vi "CellVolt181.vi"() -> ()   [LabVIEW 2018]
panel:
  in  "Boolean 15":bool
  in  "Boolean 14":bool
  in  "Boolean 13":bool
  in  "Boolean 12":bool
  in  "Table Control 15":string[][](table)=[["", "", "", "111"], ["", "", "", "112"], ["", "", "", "113"], ["", "", "", "114"], ["", "", "", "115"], ["", "", "", "116"], ["", "", "", "117"], ["", "", "", "118"], ["", "", "", "119"], ["", "", "", "120"], ["", "", "", "11"], ["", "", "", "12"], ["", "", "", "13"], ["", "", "", "14"], ["", "", "", "15"], ["", "", "", "16"], ["", "", "", "17"], ["", "", "", "18"], ["", "", "", "19"], ["", "", "", "20"], ["", "", "", "21"], ["", "", "", "22"], ["", "", "", "23"], ["", "", "", "24"]]
  in  "Table Control 14":string[][](table)=[["", "", "", "101"], ["", "", "", "102"], ["", "", "", "103"], ["", "", "", "104"], ["", "", "", "105"], ["", "", "", "106"], ["", "", "", "107"], ["", "", "", "108"], ["", "", "", "109"], ["", "", "", "110"], ["", "", "", "11"], ["", "", "", "12"], ["", "", "", "13"], ["", "", "", "14"], ["", "", "", "15"], ["", "", "", "16"], ["", "", "", "17"], ["", "", "", "18"], ["", "", "", "19"], ["", "", "", "20"], ["", "", "", "21"], ["", "", "", "22"], ["", "", "", "23"], ["", "", "", "24"]]
  in  "Table Control 13":string[][](table)=[["", "", "", "91"], ["", "", "", "92"], ["", "", "", "93"], ["", "", "", "94"], ["", "", "", "95"], ["", "", "", "96"], ["", "", "", "97"], ["", "", "", "98"], ["", "", "", "99"], ["", "", "", "100"], ["", "", "", "11"], ["", "", "", "12"], ["", "", "", "13"], ["", "", "", "14"], ["", "", "", "15"], ["", "", "", "16"], ["", "", "", "17"], ["", "", "", "18"], ["", "", "", "19"], ["", "", "", "20"], ["", "", "", "21"], ["", "", "", "22"], ["", "", "", "23"], ["", "", "", "24"]]
  in  "Table Control 12":string[][](table)=[["", "", "", "81"], ["", "", "", "82"], ["", "", "", "83"], ["", "", "", "84"], ["", "", "", "85"], ["", "", "", "86"], ["", "", "", "87"], ["", "", "", "88"], ["", "", "", "89"], ["", "", "", "90"], ["", "", "", "11"], ["", "", "", "12"], ["", "", "", "13"], ["", "", "", "14"], ["", "", "", "15"], ["", "", "", "16"], ["", "", "", "17"], ["", "", "", "18"], ["", "", "", "19"], ["", "", "", "20"], ["", "", "", "21"], ["", "", "", "22"], ["", "", "", "23"], ["", "", "", "24"]]
  in  "Table Control 11":string[][](table)=[["", "", "", "71"], ["", "", "", "72"], ["", "", "", "73"], ["", "", "", "74"], ["", "", "", "75"], ["", "", "", "76"], ["", "", "", "77"], ["", "", "", "78"], ["", "", "", "79"], ["", "", "", "80"], ["", "", "", "11"], ["", "", "", "12"], ["", "", "", "13"], ["", "", "", "14"], ["", "", "", "15"], ["", "", "", "16"], ["", "", "", "17"], ["", "", "", "18"], ["", "", "", "19"], ["", "", "", "20"], ["", "", "", "21"], ["", "", "", "22"], ["", "", "", "23"], ["", "", "", "24"]]
  in  "Boolean 10":bool
  in  "Boolean 9":bool
  in  "Boolean 8":bool
  in  "Boolean 7":bool
  in  "Boolean 6":bool
  in  "Boolean 5":bool
  in  "Table Control 10":string[][](table)=[["217"], ["218"], ["219"], ["220"], ["221"], ["222"], ["223"], ["224"], ["225"], ["226"], ["227"], ["228"], ["229"], ["230"], ["231"], ["232"], ["233"], ["234"], ["235"], ["236"], ["237"], ["238"], ["239"], ["240"]]
  in  "Table Control 9":string[][](table)=[["", "", "", "193", "", "", "", "", "", "", "193"], ["", "", "", "194", "", "", "", "", "", "", "194"], ["", "", "", "195", "", "", "", "", "", "", "195"], ["", "", "", "196", "", "", "", "", "", "", "196"], ["", "", "", "197", "", "", "", "", "", "", "197"], ["", "", "", "198", "", "", "", "", "", "", "198"], ["", "", "", "199", "", "", "", "", "", "", "199"], ["", "", "", "", "", "", "", "", "", "", "200"], ["", "", "", "", "", "", "", "", "", "", "201"], ["", "", "", "", "", "", "", "", "", "", "202"], ["", "", "", "", "", "", "", "", "", "", "203"], ["", "", "", "", "", "", "", "", "", "", "204"], ["", "", "", "", "", "", "", "", "", "", "205"], ["", "", "", "", "", "", "", "", "", "", "206"], ["", "", "", "", "", "", "", "", "", "", "207"], ["", "", "", "", "", "", "", "", "", "", "208"], ["", "", "", "", "", "", "", "", "", "", "209"], ["", "", "", "", "", "", "", "", "", "", "210"], ["", "", "", "", "", "", "", "", "", "", "211"], ["", "", "", "", "", "", "", "", "", "", "212"], ["", "", "", "", "", "", "", "", "", "", "213"], ["", "", "", "", "", "", "", "", "", "", "214"], ["", "", "", "", "", "", "", "", "", "", "215"], ["", "", "", "", "", "", "", "", "", "", "216"]]
  in  "Table Control 8":string[][](table)=[["", "", "", "169"], ["", "", "", "170"], ["", "", "", "171"], ["", "", "", "172"], ["", "", "", "173"], ["", "", "", "174"], ["", "", "", "175"], ["", "", "", "176"], ["", "", "", "177"], ["", "", "", "175"], ["", "", "", "179"], ["", "", "", "180"], ["", "", "", "181"], ["", "", "", "182"], ["", "", "", "183"], ["", "", "", "184"], ["", "", "", "185"], ["", "", "", "186"], ["", "", "", "187"], ["", "", "", "188"], ["", "", "", "189"], ["", "", "", "190"], ["", "", "", "191"], ["", "", "", "192"]]
  in  "Table Control 7":string[][](table)=[["", "", "", "145"], ["", "", "", "146"], ["", "", "", "147"], ["", "", "", "148"], ["", "", "", "149"], ["", "", "", "150"], ["", "", "", "151"], ["", "", "", "152"], ["", "", "", "153"], ["", "", "", "154"], ["", "", "", "155"], ["", "", "", "156"], ["", "", "", "157"], ["", "", "", "158"], ["", "", "", "159"], ["", "", "", "160"], ["", "", "", "161"], ["", "", "", "162"], ["", "", "", "163"], ["", "", "", "164"], ["", "", "", "165"], ["", "", "", "166"], ["", "", "", "167"], ["", "", "", "168"]]
  in  "Table Control 6":string[][](table)=[["", "", "", "121"], ["", "", "", "122"], ["", "", "", "123"], ["", "", "", "124"], ["", "", "", "125"], ["", "", "", "126"], ["", "", "", "127"], ["", "", "", "128"], ["", "", "", "129"], ["", "", "", "130"], ["", "", "", "131"], ["", "", "", "132"], ["", "", "", "133"], ["", "", "", "134"], ["", "", "", "135"], ["", "", "", "136"], ["", "", "", "137"], ["", "", "", "138"], ["", "", "", "139"], ["", "", "", "140"], ["", "", "", "141"], ["", "", "", "142"], ["", "", "", "143"], ["", "", "", "144"], ["", "", "", "145"]]
  in  "Table Control 5":string[][](table)=[["", "", "", "97"], ["", "", "", "98"], ["", "", "", "99"], ["", "", "", "100"], ["", "", "", "101"], ["", "", "", "102"], ["", "", "", "103"], ["", "", "", "104"], ["", "", "", "105"], ["", "", "", "106"], ["", "", "", "107"], ["", "", "", "108"], ["", "", "", "109"], ["", "", "", "110"], ["", "", "", "111"], ["", "", "", "112"], ["", "", "", "113"], ["", "", "", "114"], ["", "", "", "115"], ["", "", "", "116"], ["", "", "", "117"], ["", "", "", "118"], ["", "", "", "119"], ["", "", "", "120"]]
  in  "Table Control 4":string[][](table)=[["", "", "", "73"], ["", "", "", "74"], ["", "", "", "75"], ["", "", "", "76"], ["", "", "", "77"], ["", "", "", "78"], ["", "", "", "79"], ["", "", "", "80"], ["", "", "", "81"], ["", "", "", "82"], ["", "", "", "83"], ["", "", "", "84"], ["", "", "", "85"], ["", "", "", "86"], ["", "", "", "87"], ["", "", "", "88"], ["", "", "", "89"], ["", "", "", "90"], ["", "", "", "91"], ["", "", "", "92"], ["", "", "", "93"], ["", "", "", "94"], ["", "", "", "95"], ["", "", "", "96"], ["", "", "", "97"]]
  in  "Table Control 3":string[][](table)=[["", "", "", "49"], ["", "", "", "50"], ["", "", "", "51"], ["", "", "", "52"], ["", "", "", "53"], ["", "", "", "54"], ["", "", "", "55"], ["", "", "", "56"], ["", "", "", "57"], ["", "", "", "58"], ["", "", "", "59"], ["", "", "", "60"], ["", "", "", "61"], ["", "", "", "62"], ["", "", "", "63"], ["", "", "", "64"], ["", "", "", "65"], ["", "", "", "66"], ["", "", "", "67"], ["", "", "", "68"], ["", "", "", "69"], ["", "", "", "70"], ["", "", "", "71"], ["", "", "", "72"], ["", "", "", "73"]]
  in  "Table Control 2":string[][](table)=[["", "", "", "25"], ["", "", "", "26"], ["", "", "", "27"], ["", "", "", "28"], ["", "", "", "29"], ["", "", "", "30"], ["", "", "", "31"], ["", "", "", "32"], ["", "", "", "33"], ["", "", "", "34"], ["", "", "", "35"], ["", "", "", "36"], ["", "", "", "37"], ["", "", "", "38"], ["", "", "", "39"], ["", "", "", "40"], ["", "", "", "41"], ["", "", "", "42"], ["", "", "", "43"], ["", "", "", "44"], ["", "", "", "45"], ["", "", "", "46"], ["", "", "", "47"], ["", "", "", "48"]]
  in  "Table Control":string[][](table)=[["", "", "", "61"], ["", "", "", "62"], ["", "", "", "63"], ["", "", "", "64"], ["", "", "", "65"], ["", "", "", "66"], ["", "", "", "67"], ["", "", "", "68"], ["", "", "", "69"], ["", "", "", "70"], ["", "", "", "11"], ["", "", "", "12"], ["", "", "", "13"], ["", "", "", "14"], ["", "", "", "15"], ["", "", "", "16"], ["", "", "", "17"], ["", "", "", "18"], ["", "", "", "19"], ["", "", "", "20"], ["", "", "", "21"], ["", "", "", "22"], ["", "", "", "23"], ["", "", "", "24"]]
  in  "Boolean 4":bool
  in  "Boolean 3":bool
  in  "Boolean 2":bool
  in  "Boolean":bool
  # "BMS Monitor"
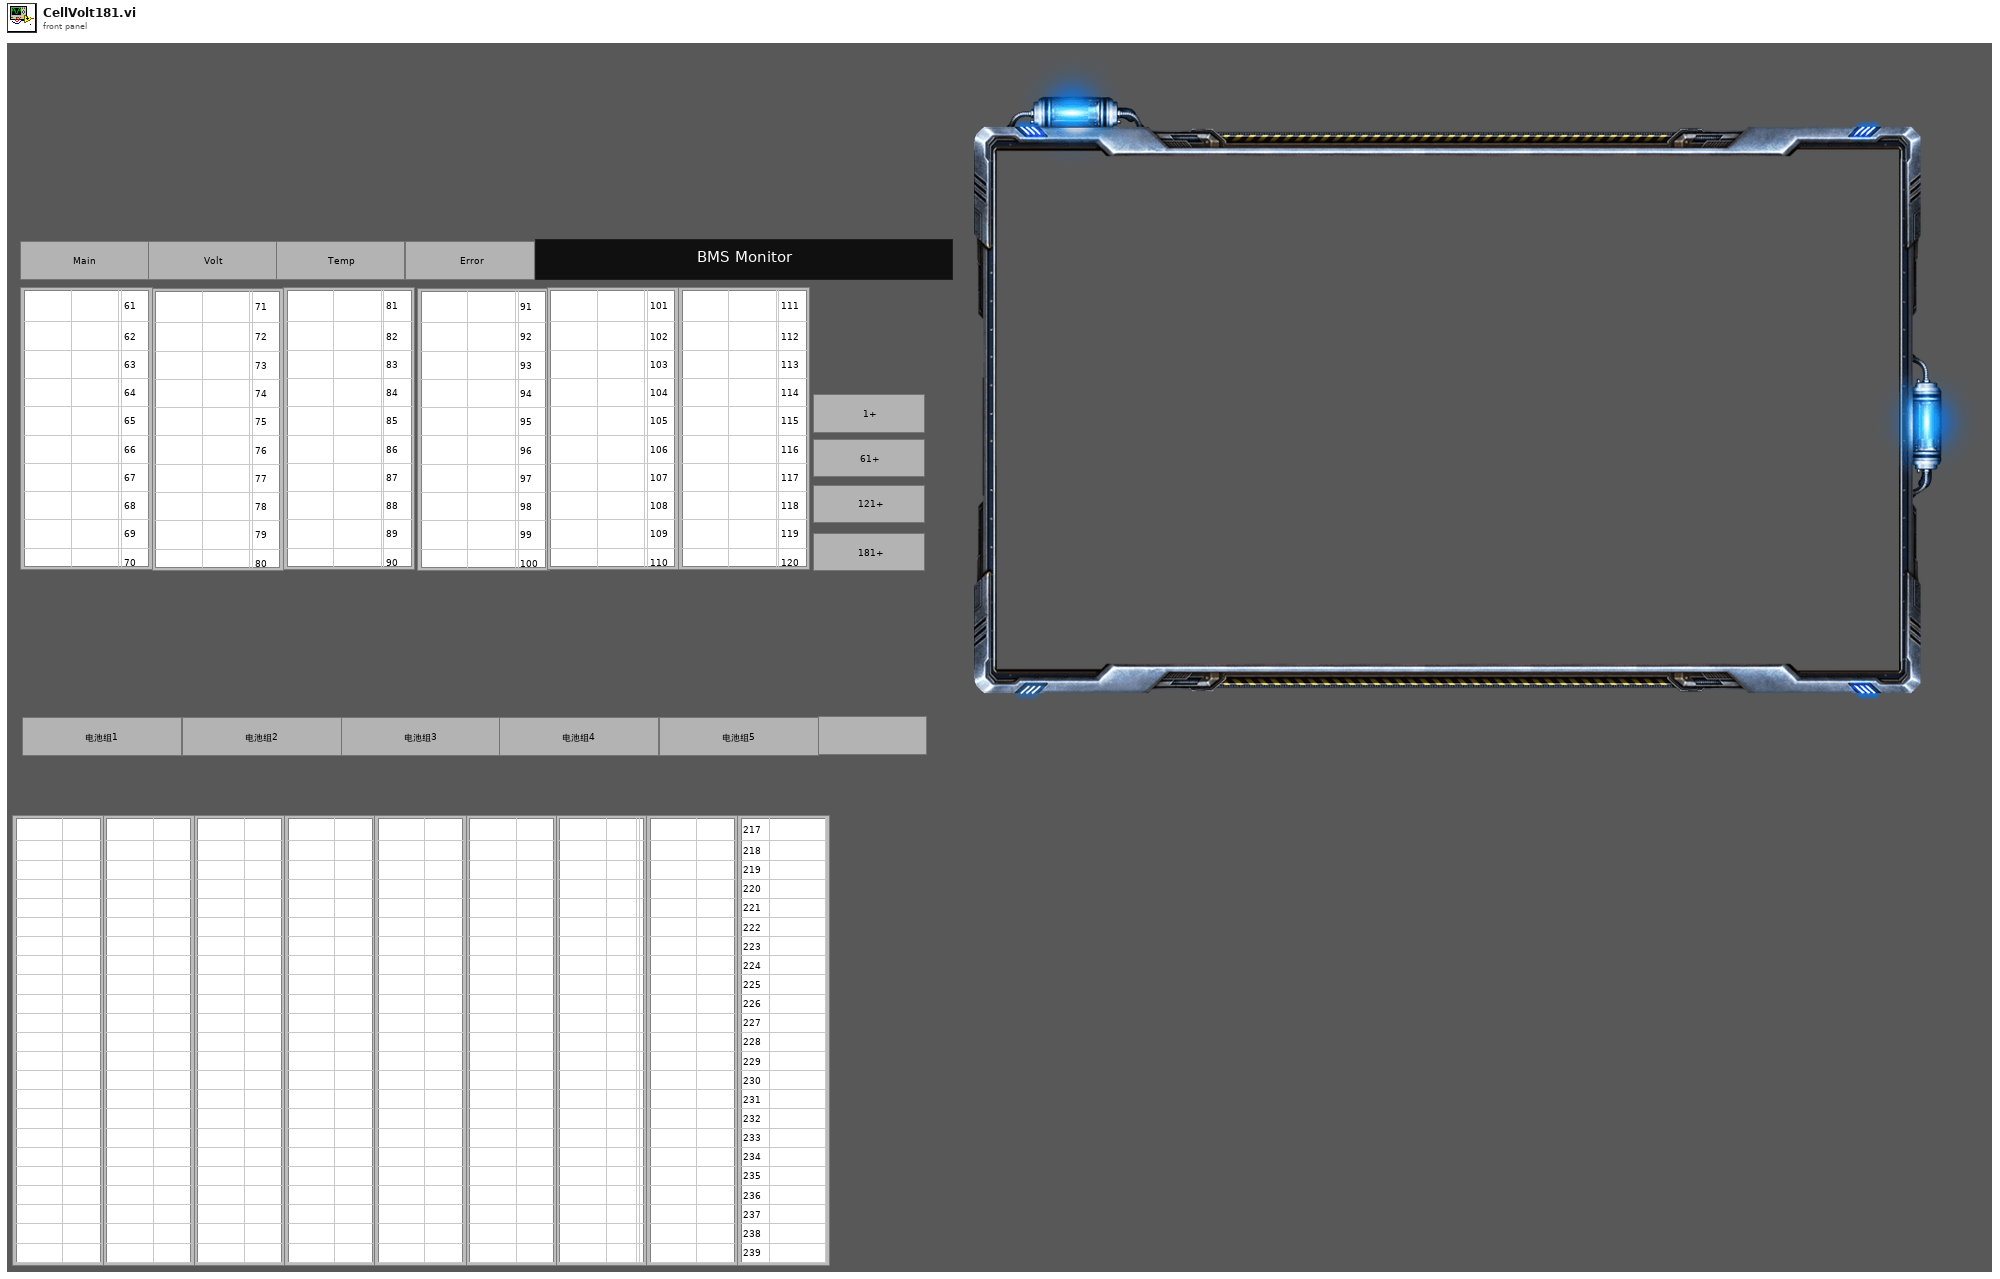
[diagram p1: front panel]
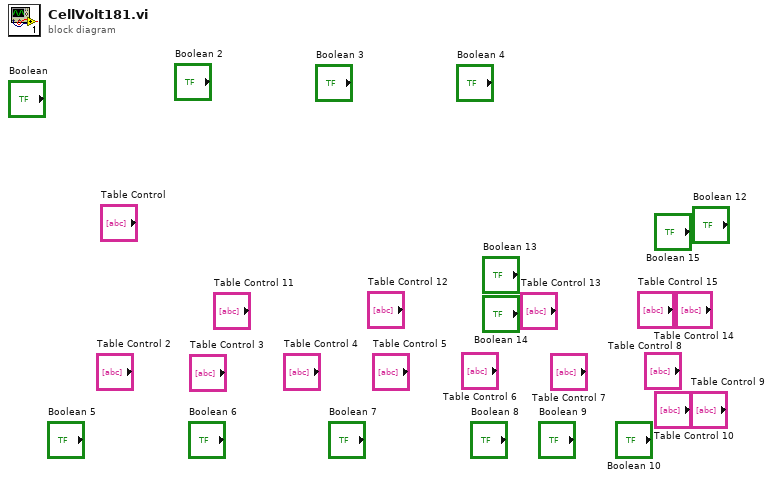
[diagram p0: block diagram]
diagram:
